vi "Pose.vi"() -> ()   [LabVIEW 2015]
panel:
  out "Waveform Chart":dbl(graph)
  in  "String":string
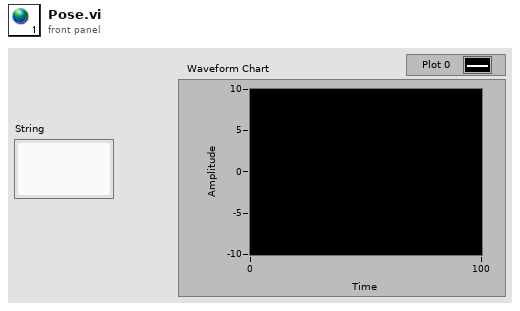
[diagram p1: front panel]
diagram:
